vi "Autonomous Independent.vi"   [LabVIEW 2017]
doc: "This VI is called when autonomous begins, and will automatically be terminated when autonomous ends. You can carry out timed or sensor driven robot movement independently without needing to return to the caller."
uses:
  <vilib>/Rock Robotics/Network Tables/NT Write String.vi
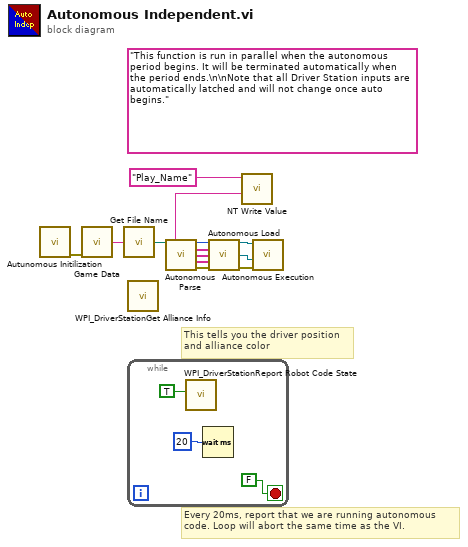
[diagram p0: block diagram]
diagram:
  (unwired) "This function is run in parallel when the autonomous period begins. It will be terminated automatically when the period ends.\n\nNote that all Driver Station inputs are automatically latched and will not change once auto begins."
  # "Every 20ms, report that we are running autonomous\ncode. Loop will abort the same time as the VI."
  # "This tells you the driver position\nand alliance color"
  n1 = call "Autunomous Initilization.vi"() -> ("errror out"=w5:errorcluster)  [unwired: 11 in]
  n2 = call "Game Data.vi"("error in"=w5) -> ("Game Specific Data"=w2:string)  [unwired: 5 in]
  n3 = call "Get File Name.vi"("Game Data"=w2) -> ("File Name"=w1:path)
  n4 = call <vilib>:"WPI_DriverStationGet Alliance Info.vi"() -> ()  [unwired: 12 out]
  n5 = while {
    stop <- FALSE stop-if-true
    n6 = call <vilib>:"WPI_DriverStationReport Robot Code State.vi"("Autonomous"=TRUE) -> ()  [unwired: 10 in, 1 out]
    n7 = Wait (ms)(milliseconds to wait=u32 20) -> ()  [unwired: 1 out]
  }
  n8 = call "Autonomous Parse.vi"("File Path"=w1) -> ("Name of Play"=w4:string, "Number of Commands"=w8:i32, "Subsystems"=w6:string[], "Commands"=w7:string[], "Inputs"=w9:string[], "errror out"=w13:errorcluster)  [unwired: 8 in, 1 out]
  n9 = call "Autonomous Load.vi"("Number of Commands"=w8, "Subsystems"=w6, "Commands"=w7, "Inputs"=w9, "error in"=w13) -> ("Queue Key"=w11:refnum<queue>, "Autonomous Queue"=w10:refnum<queue>, "errror out"=w12:errorcluster)  [unwired: 7 in, 1 out]
  n10 = call-poly <vilib>:"NT Write Value.vi"("String"=w4, "Name"="Play_Name") -> ()  [unwired: 9 in, 1 out]
  n11 = call "Autonomous Execution.vi"("error in"=w12, "Autonomous Queue"=w10, "Queue Key"=w11) -> ()  [unwired: 9 in]
